vi "Configure Marker Reflection Measurement.vi"(7 "Enable Continuous Peak (F: Disable)":bool, 8 "error in (no error)":errorcluster, 9 "Enable Continuous Valley (F: Disable)":bool, 10 "Active Marker (1: Marker 1)":i32(ring)=1 items=["Marker 1"=1, "Marker 2"=2, "Marker 3"=3, "Marker 4"=4, "Marker 5"=5, "Marker 6"=6], 11 "VISA resource name":refnum<visa-resource-name>) -> (0 "error out":errorcluster, 3 "VISA resource name out":refnum<visa-resource-name>)   [LabVIEW 2022 SP3, in "Agilent N934X Series.lvlib"]
doc: "Configures the marker state of Reflection Measurement Option.\n\nNote:\nThis VI is only applicable for N9321C, N9322C, N9323C, N9324C models."
uses:
  <instrlib>/Agilent N934X Series/Agilent N934X Series.lvlib
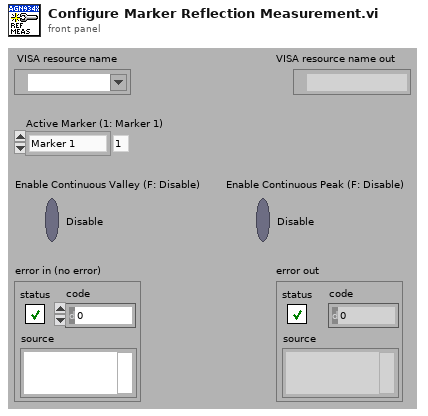
[diagram p1: front panel]
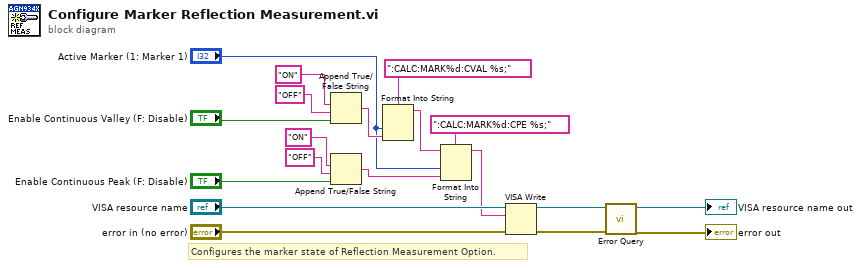
[diagram p0: block diagram]
diagram:
  # "Configures the marker state of Reflection Measurement Option."
  n1 = Append True/False String(1:"Enable Continuous Valley (F: Disable)", 2:"OFF", 3:"ON") -> (0:w15:string)  [unwired: 1 in]
  n2 = Append True/False String(1:"Enable Continuous Peak (F: Disable)", 2:"OFF", 3:"ON") -> (0:w4:string)  [unwired: 1 in]
  n3 = Format Into String(format string=":CALC:MARK%d:CVAL %s;", "Active Marker (1: Marker 1)", w15) -> (resulting string=w6:string)  [unwired: 2 in, 1 out]
  n4 = Format Into String(format string=":CALC:MARK%d:CPE %s;", initial string=w6, "Active Marker (1: Marker 1)", w4) -> (resulting string=w3:string)  [unwired: 1 in, 1 out]
  n5 = VISA Write(VISA resource name="VISA resource name", write buffer=w3, error in (no error)="error in (no error)") -> (VISA resource name out=w12:refnum<visa-resource-name>, error out=w11:errorcluster)  [unwired: 1 out]
  n6 = call <instrlib>:"Error Query.vi"("error in (no error)"=w11, "VISA resource name"=w12) -> ("error out"=→"error out":errorcluster, "VISA resource name out"=→"VISA resource name out":refnum<visa-resource-name>)  [unwired: 6 in, 2 out]
